vi "Read Nest Actor Aliases.vi"(7 "Self Actor":refnum<class "LVCAM.lvclass">, 10 "Alias":string) -> (0 "error out":errorcluster, 1 "Alias found?":bool, 2 "Nest Actor Aliases":string[](array[string]))   [LabVIEW 2021, in "LVCAM.lvlib" / "Self Actor.lvclass"]
uses:
  Self Actor.lvclass
  LVCAM/LVCAM.lvclass
  Self Actor.lvclass/Self Actor.ctl
  Msg Q/Msg Q.lvclass
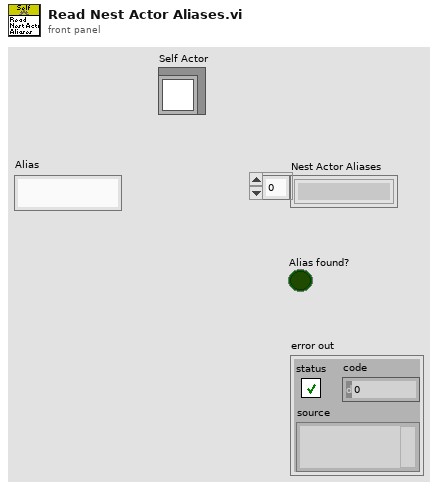
[diagram p1: front panel]
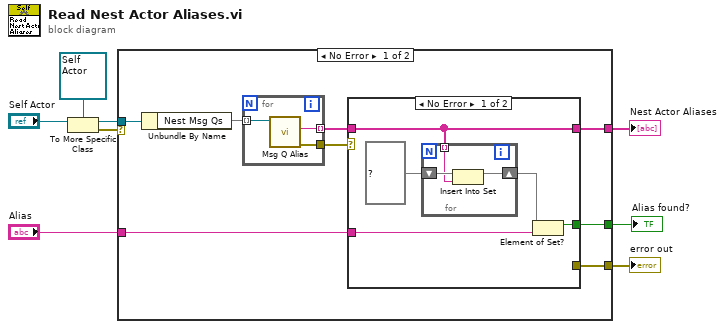
[diagram p0: block diagram]
diagram:
  n1 = To More Specific Class(target class=refnum<class "Self Actor.lvclass"> refnum ("LVCAM.lvlib:Self Actor.lvclass"), reference="Self Actor") -> (specific class reference=w5:refnum<class "Self Actor.lvclass">, error out=w3:errorcluster)  [unwired: 1 in]
  n2 = case shown="No Error" w3 {
    selector: w3 -> [_ w29]
    tunnel: [w13 w29] -> w8
    tunnel: [w12 _] -> w7
    tunnel: w5 -> [w15 _]
    tunnel: "Alias" -> [w10 _]
    tunnel: [w9 _] -> w1
    frame No Error {
      n3 = Unbundle By Name(w15) -> ("Nest Msg Qs"=w16:set{refnum<class "Msg Q.lvclass">})
      n4 = for {
        tunnel: w16 -> [w28] mode=indexing
        tunnel: [w27] -> w11 mode=indexing
        tunnel: [w26] -> w14
        n5 = call "Msg Q Alias.vi"("Msg Q in"=w28) -> ("error out"=w26:errorcluster, "Msg Q Alias"=w27:string)  [unwired: 9 in]
      }
      n6 = case shown="No Error" w14 {
        selector: w14 -> [_ w25]
        tunnel: [_ w25] -> w13
        tunnel: [w18 _] -> w12
        tunnel: w11 -> [w18 _]
        tunnel: w10 -> [w19 _]
        tunnel: [w17 _] -> w9
        frame No Error {
          n7 = for {
            tunnel: w18 -> [w22] mode=indexing
            shift-right: [w24] -> w20
            shift-left: set{string} {} ("empty set") -> [w23]
            n8 = Insert Into Set(10:w22, 11:w23) -> (3:w24:set{string})  [unwired: 1 out]
          }
          n9 = Element of Set?(10:w19, 11:w20) -> (3:w17:bool)
        }
        frame Error {
          # "#LVCAMError"
        }
      }
    }
    frame Error {
    }
  }
  "error out" <- w8
  "Nest Actor Aliases" <- w7
  "Alias found?" <- w1
